vi "Receive Message.vi"(6 "priority":i32, 10 "IMediator in":refnum<class "IMediator.lvclass">, 11 "Message in":refnum<class "Message.lvclass">) -> (0 "error out":errorcluster, 2 "Actor out":refnum<class "Actor.lvclass">)   [LabVIEW 2017, in "IMediator.lvlib" / "IMediator.lvclass"]
doc: "This VI should be overriden ONLY if you are creating a proxy actor for remote transmission. If you are, override this VI to transmit the received message to a new destination, maintaining the given priority."
uses:
  IMediator.lvclass
  gpm_packages/@cs/event-logger/Source/Composed Log/Composed Log.lvlib
  gpm_packages/@cs/event-logger/Source/Composed Log/Log Sink/Log Level.ctl
  gpm_packages/@cs/event-logger/Source/Composed Log/Log Sink/Log Sink.lvclass
  IMediator Messages/Publish Msg/Publish Msg.lvclass
  <vilib>/ActorFramework/Actor/Actor.lvclass
  <vilib>/ActorFramework/Message/Message.lvclass
  C:/Program Files (x86)/National Instruments/LabVIEW 2017/vi.lib/ActorFramework/Actor/Actor.lvclass
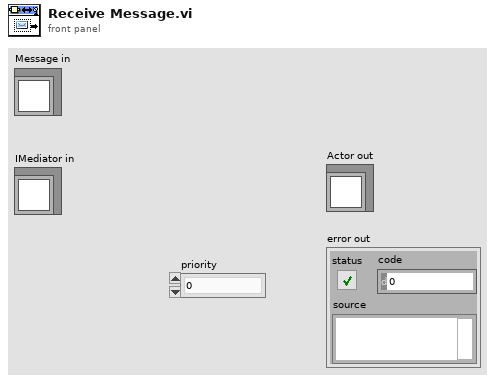
[diagram p1: front panel]
types:
  T1 = typedef "Composed Log.lvlib/Log Sink.lvclass/Log Level.ctl" = enum16{"Debug", "Info", "Warning", "Error", "Critical"}
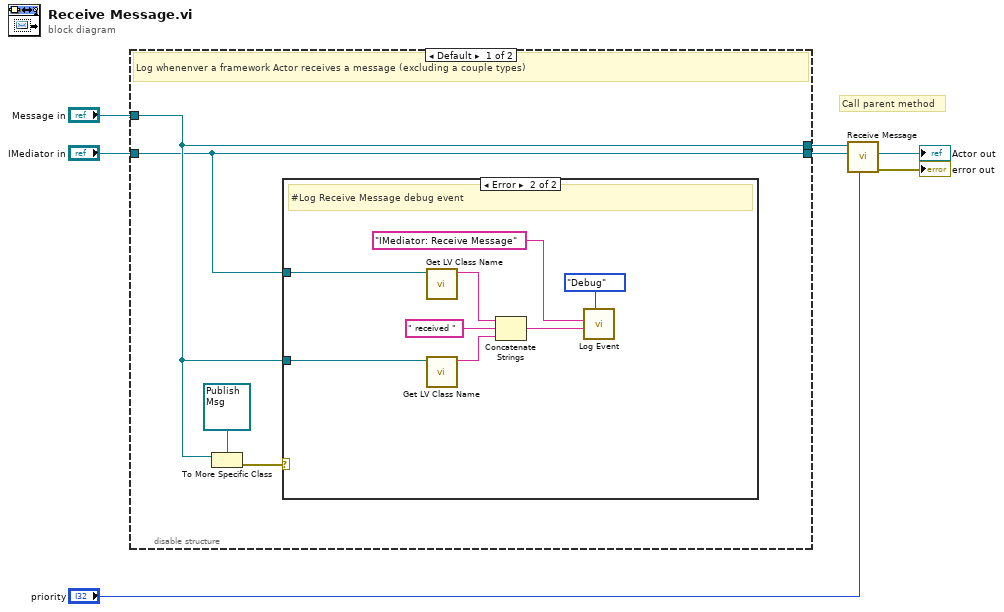
[diagram p0: block diagram]
diagram:
  # "Call parent method"
  n1 = disable-structure shown="Default" {
    disable-tunnel: "Message in" -> [w11 w21]
    disable-tunnel: "IMediator in" -> [w10 w20]
    disable-tunnel: [w11 w21] -> w2
    disable-tunnel: [w10 w20] -> w1
    frame condition #0 (active) {
      # "Log whenenver a framework Actor receives a message (excluding a couple types)"
      n2 = To More Specific Class(target class=refnum<class "Publish Msg.lvclass"> refnum ("IMediator.lvlib:Publish Msg.lvclass"), reference=w11) -> (error out=w8:errorcluster)  [unwired: 1 in, 1 out]
      n3 = case shown="Error" w8 {
        tunnel: w11 -> [_ w15]
        tunnel: w10 -> [_ w14]
        frame No Error {
          # "Exclude logging for mediated datum updates\nbecause there. are. just. too. many. of. them."
          # "Message is a Publish Msg -- Do not log this message type"
        }
        frame Error {
          # "#Log Receive Message debug event"
          n4 = call <vilib>:"Get LV Class Name.vi"("object"=w14) -> ("class name"=w16:string)  [unwired: 9 in, 1 out]
          n5 = call <vilib>:"Get LV Class Name.vi"("object"=w15) -> ("class name"=w17:string)  [unwired: 9 in, 1 out]
          n6 = Concatenate Strings(w16, " received " ("string"), w17) -> (w12:string)
          n7 = call "Log Event.vi"("Event Level"=Log_Level."Debug", "Data To Log"=w12, "SourceID"="IMediator: Receive Message") -> ()  [unwired: 7 in, 2 out]
        }
      }
    }
    frame condition #1 {
      # "Remove all logging from this method at compile time"
    }
  }
  n8 = call-parent "Receive Message.vi"("priority"="priority", "Actor in"=w1, "Message in"=w2) -> ("error out"=→"error out":errorcluster, "Actor out"=→"Actor out":refnum<class "Actor.lvclass">)  [unwired: 7 in]
